vi "Write Reason.vi"(8 "error in (no error)":errorcluster, 10 "Reason":errorcluster, 11 "Rejected Future in":refnum<class "Rejected Promise.lvclass">) -> (0 "error out":errorcluster, 3 "Rejected Future out":refnum<class "Rejected Promise.lvclass">)   [LabVIEW 2017, in "Promise.lvlib" / "Rejected Promise.lvclass"]
uses:
  Rejected Promise.lvclass
  Rejected Promise.lvclass/Rejected Promise.ctl
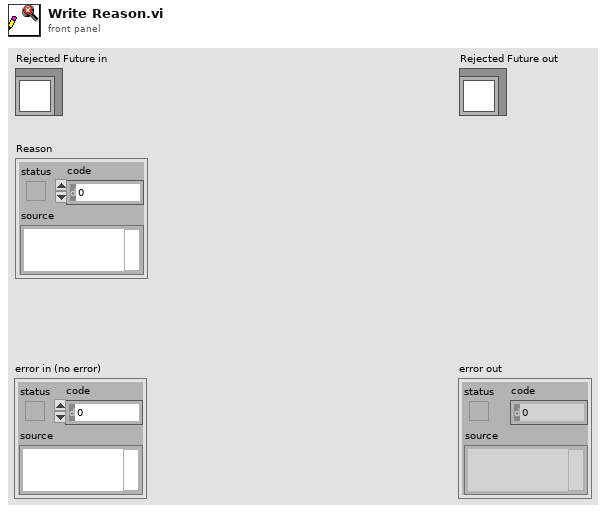
[diagram p1: front panel]
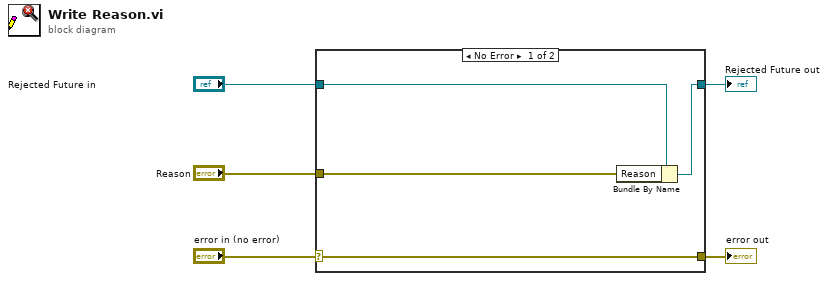
[diagram p0: block diagram]
diagram:
  n1 = case shown="No Error" "error in (no error)" {
    selector: "error in (no error)" -> [w9 w10]
    tunnel: [w9 w10] -> w4
    tunnel: [w7 w11] -> w2
    tunnel: "Rejected Future in" -> [w8 w11]
    tunnel: "Reason" -> [w6 _]
    frame No Error {
      n2 = Bundle By Name(cluster=w8, "Reason"=w6) -> (w7:refnum<class "Rejected Promise.lvclass">)
    }
    frame Error {
    }
  }
  "error out" <- w4
  "Rejected Future out" <- w2
